vi "harvard_pump_test.vi"() -> ()   [LabVIEW 2014]
uses:
  <vilib>/Instr/_visa.llb/VISA Configure Serial Port (Instr).vi
panel:
  in  "Sample Channel\nFlow":bool
  out "error out":errorcluster
  in  "Stop Flow":bool
  in  "Start Flow":bool
  in  "stop":bool
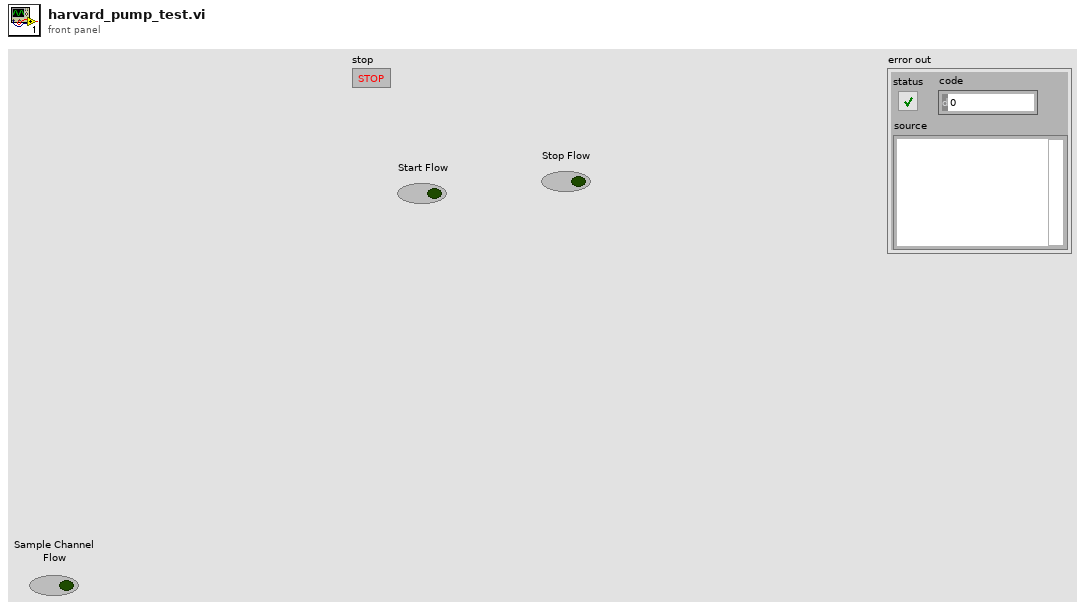
[diagram p1: front panel]
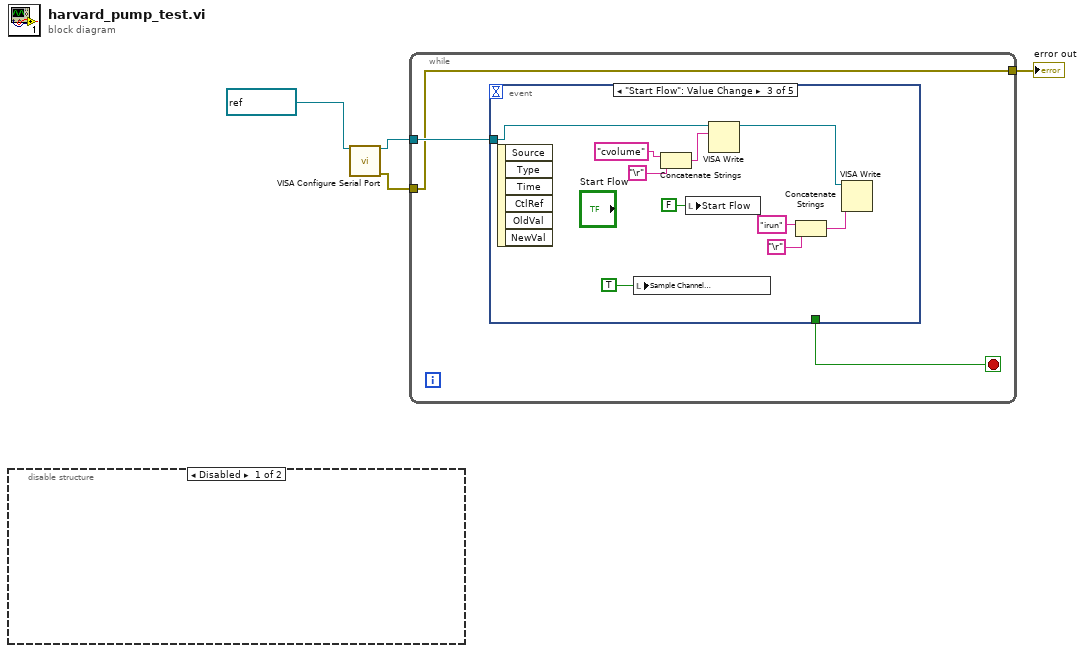
[diagram p0: block diagram]
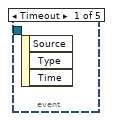
[diagram p3: hidden frame]
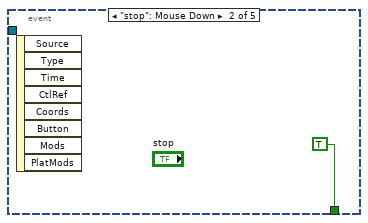
[diagram p4: hidden frame]
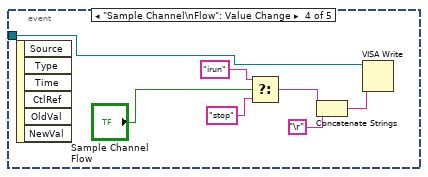
[diagram p5: hidden frame]
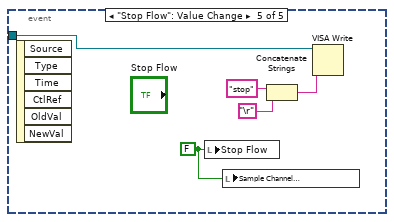
[diagram p6: hidden frame]
diagram:
  n1 = disable-structure shown="Disabled" {
    frame Disabled {
    }
    frame Enabled {
    }
  }
  n2 = call-poly "VISA Configure Serial Port"("VISA resource name"=refnum<visa-resource-name> "COM2") -> ("VISA resource name out"=w1:refnum<visa-resource-name>, "error out"=w4:errorcluster)  [unwired: 5 in, 8 out]
  n3 = while {
    tunnel: w1 -> [w6]
    tunnel: w4 -> [w5]
    tunnel: [w5] -> w3
    stop <- w7 stop-if-true
    n4 = event shown="[2] \"Start Flow\": Value Change" {
      selector: _ -> [_ _ _ _ _]
      dyn-events: _ -> [_ _ _ _ _]
      timeout: _ -> [_ _ _ _ _]
      tunnel: [_ TRUE _ _ _] -> w7
      tunnel: w6 -> [_ _ w10 w19 w27]
      event Timeout {
        n5 = event-data() -> ()  [unwired: 1 in, 3 out]
      }
      event "stop": Mouse Down {
        n6 = event-data() -> ()  [unwired: 1 in, 8 out]
      }
      event "Start Flow": Value Change {
        n7 = event-data() -> ()  [unwired: 1 in, 6 out]
        n8 = local write "Sample Channel\nFlow"(TRUE ("Sample Channel\nFlow")) -> ()
        n9 = Concatenate Strings("cvolume" ("string"), "\r") -> (w11:string)
        n10 = local write "Start Flow"(FALSE ("Start Flow")) -> ()
        n11 = VISA Write(VISA resource name=w10, write buffer=w11) -> (VISA resource name out=w9:refnum<visa-resource-name>)  [unwired: 1 in, 2 out]
        n12 = Concatenate Strings("irun" ("string"), "\r") -> (w16:string)
        n13 = VISA Write(VISA resource name=w9, write buffer=w16) -> ()  [unwired: 1 in, 3 out]
      }
      event "Sample Channel\nFlow": Value Change {
        n14 = event-data() -> ()  [unwired: 1 in, 6 out]
        n15 = Select(t="irun" ("string"), s="Sample Channel\nFlow", f="stop" ("string")) -> (s? t:f=w24:string)
        n16 = Concatenate Strings(w24, "\r") -> (w21:string)
        n17 = VISA Write(VISA resource name=w19, write buffer=w21) -> ()  [unwired: 1 in, 3 out]
      }
      event "Stop Flow": Value Change {
        w26 = FALSE ("Stop Flow")
        n18 = event-data() -> ()  [unwired: 1 in, 6 out]
        n19 = local write "Stop Flow"(w26) -> ()
        n20 = local write "Sample Channel\nFlow"(w26) -> ()
        n21 = Concatenate Strings("stop" ("string"), "\r") -> (w29:string)
        n22 = VISA Write(VISA resource name=w27, write buffer=w29) -> ()  [unwired: 1 in, 3 out]
      }
    }
  }
  "error out" <- w3
